vi "Main.vi"() -> ()   [LabVIEW 2013]
doc: "Main code that will run on the robot and contains all the logic and hardware interfaces."
uses:
  Data/TypeDefs/UTM Location.ctl
  Data/TypeDefs/Sail Set Suggestions.ctl
  Data/TypeDefs/Rudder Set Suggestions.ctl
  Data/TypeDefs/OverrideInformation.ctl
  Data/TypeDefs/OverrideMode.ctl
  Logic/Classes/Missions/GenericMission/GenericMission.lvclass
  Logic/Classes/Obstacle/Obstacle.lvclass
  Logic/Classes/Logger/Logger.lvclass
panel:
  out "appended path":path
  out "Missions":refnum<class "GenericMission.lvclass">[](array[class])
  out "Obstacles":refnum<class "Obstacle.lvclass">[](array[class])
  out "Finished Missions":refnum<class "GenericMission.lvclass">[](array[class])
  out "OverrideInformation":T1={"OverrideMode"=enum."Rudder", "SailSetting"={"MainSailSuggestion"=0.0, "JibSailSuggestion"=0.0}, "Rudder Setpoint"=0.0, "Sim_Wind_Speed"=0.0, "Sim_Wind_Heading"=0.0} {"SailSetting"."MainSailSuggestion" min=0.0 max=1.0; "SailSetting"."JibSailSuggestion" min=0.0 max=1.0; "Rudder Setpoint" min=-0.95 max=0.95 scale=1.0..-1.0}
  out "DisplayCounter":i32
  out "AbsWindDirection":dbl
  out "IronsRange":dbl
  out "RudderPosition":T4 min=-0.95 max=0.95 scale=1.0..-1.0
  out "SailPositions":T3 {"MainSailSuggestion" min=0.0 max=1.0; "JibSailSuggestion" min=0.0 max=1.0}
  out "RelWindDirection":dbl
  out "RateOfTurn":dbl
  out "BoatLocation":T5 {"North" format="%#_10f"; "East" format="%#_8f"}
  out "BoatDirection":dbl
  out "WindSpeed":dbl
  out "BoatSpeed":dbl
  in  "XBee Serial Port":refnum<visa-resource-name>="COM8"
  in  "Boat Type":T6(ring)=enum."Simulation"
  in  "stop":bool
  # "ALL THE DEBUG INFO - Eric"
  # "SET THIS BEFORE RUNNING\nOR YOU WILL NEED TO\nRESTART THE CODE!!!"
  # "For Little Boat Initialization"
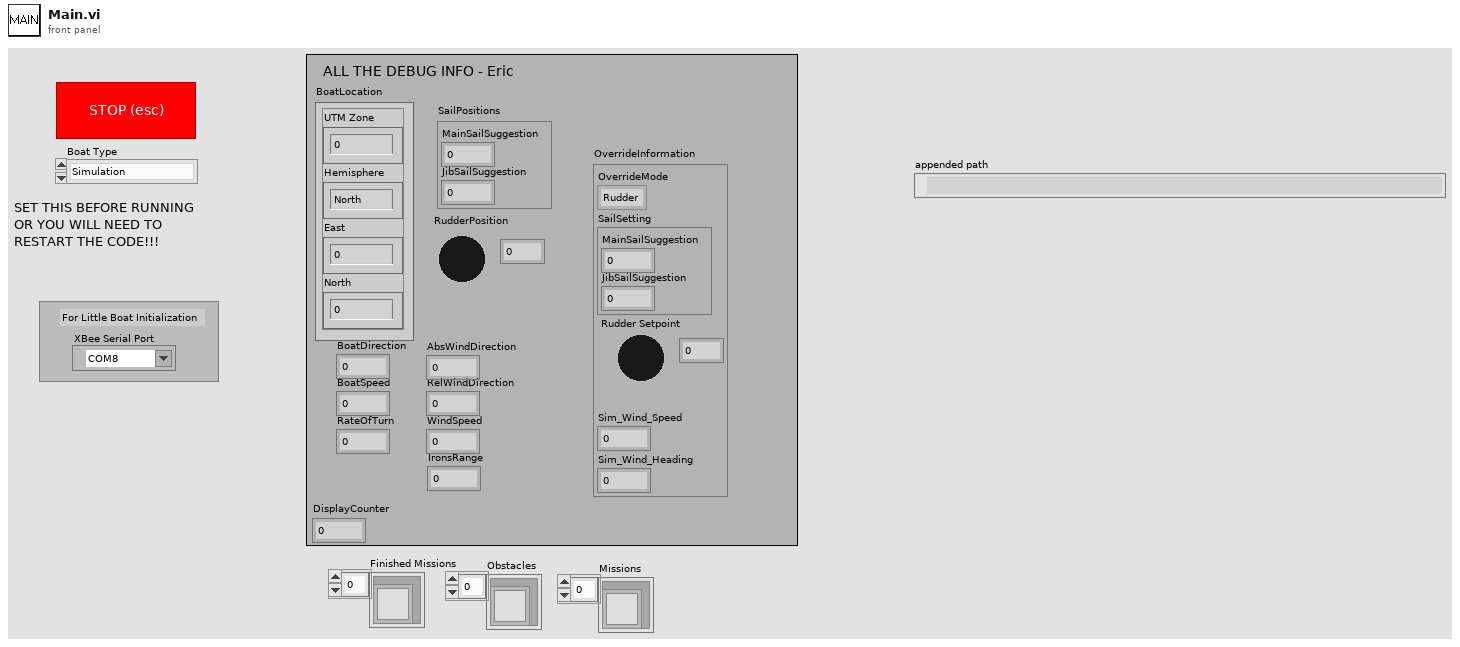
[diagram p1: front panel]
types:
  T1 = typedef "OverrideInformation.ctl" = cluster{"OverrideMode":T2, "SailSetting":T3, "Rudder Setpoint":T4, "Sim_Wind_Speed":dbl, "Sim_Wind_Heading":dbl}
  T2 = typedef "OverrideMode.ctl" = enum16{"None", "Rudder", "Sails", "Both"}
  T3 = typedef "Sail Set Suggestions.ctl" = cluster{"MainSailSuggestion":dbl, "JibSailSuggestion":dbl}
  T4 = typedef "Rudder Set Suggestions.ctl" = dbl
  T5 = typedef "UTM Location.ctl" = cluster{"UTM Zone":dbl, "Hemisphere":enum16{"North", "South"}, "East":dbl, "North":dbl}
  T6 = enum16{"Blackbody Radiation", "Little boats", "Simulation", "Damn Yankee"}
  T7 = typedef "MissionNotifiers.ctl" = cluster{"Missions":refnum<notifier>, "Finished Missions":refnum<notifier>, "Obstacles":refnum<notifier>}
  T8 = typedef "Notifiers.ctl" = cluster{"BoatSpeed":refnum<notifier>, "WindSpeed":refnum<notifier>, "EStop":refnum<notifier>, "BoatDirection":refnum<notifier>, "Luffing":refnum<notifier>, "RudderForce":refnum<notifier>, "BatteryVoltage":refnum<notifier>, "StayForces":refnum<notifier>, "BoatLocation":refnum<notifier>, "Pitch":refnum<notifier>, "Roll":refnum<notifier>, "RateOfTurn":refnum<notifier>, "RelWindDirection":refnum<notifier>, "SailPositions":refnum<notifier>, "RudderPosition":refnum<notifier>, "IronsRange":refnum<notifier>, "AbsWindDirection":refnum<notifier>, "OverrideInformation":refnum<notifier>, "DynamixelTorques":refnum<notifier>, "MotorSetup":refnum<notifier>, "AirmarStatus":refnum<notifier>, "HardwareOnline?":refnum<notifier>, "Sim_ActualSailPositions [0,1]":refnum<notifier>, "DynamixelCycleTracker":refnum<notifier>, "BoatVelocityDirection":refnum<notifier>, "SimWindHeading(rad)":refnum<notifier>, "SimWindSpeed(m/s)":refnum<notifier>, "RCInputValues":refnum<notifier>, "Finished Waypoints":refnum<notifier>, "DesiredHeading":refnum<notifier>, "Latest Mission ID":refnum<notifier>, "Latest Obstacle ID":refnum<notifier>}
  T9 = typedef "Queues.ctl" = cluster{"Waypoints":refnum<queue>}
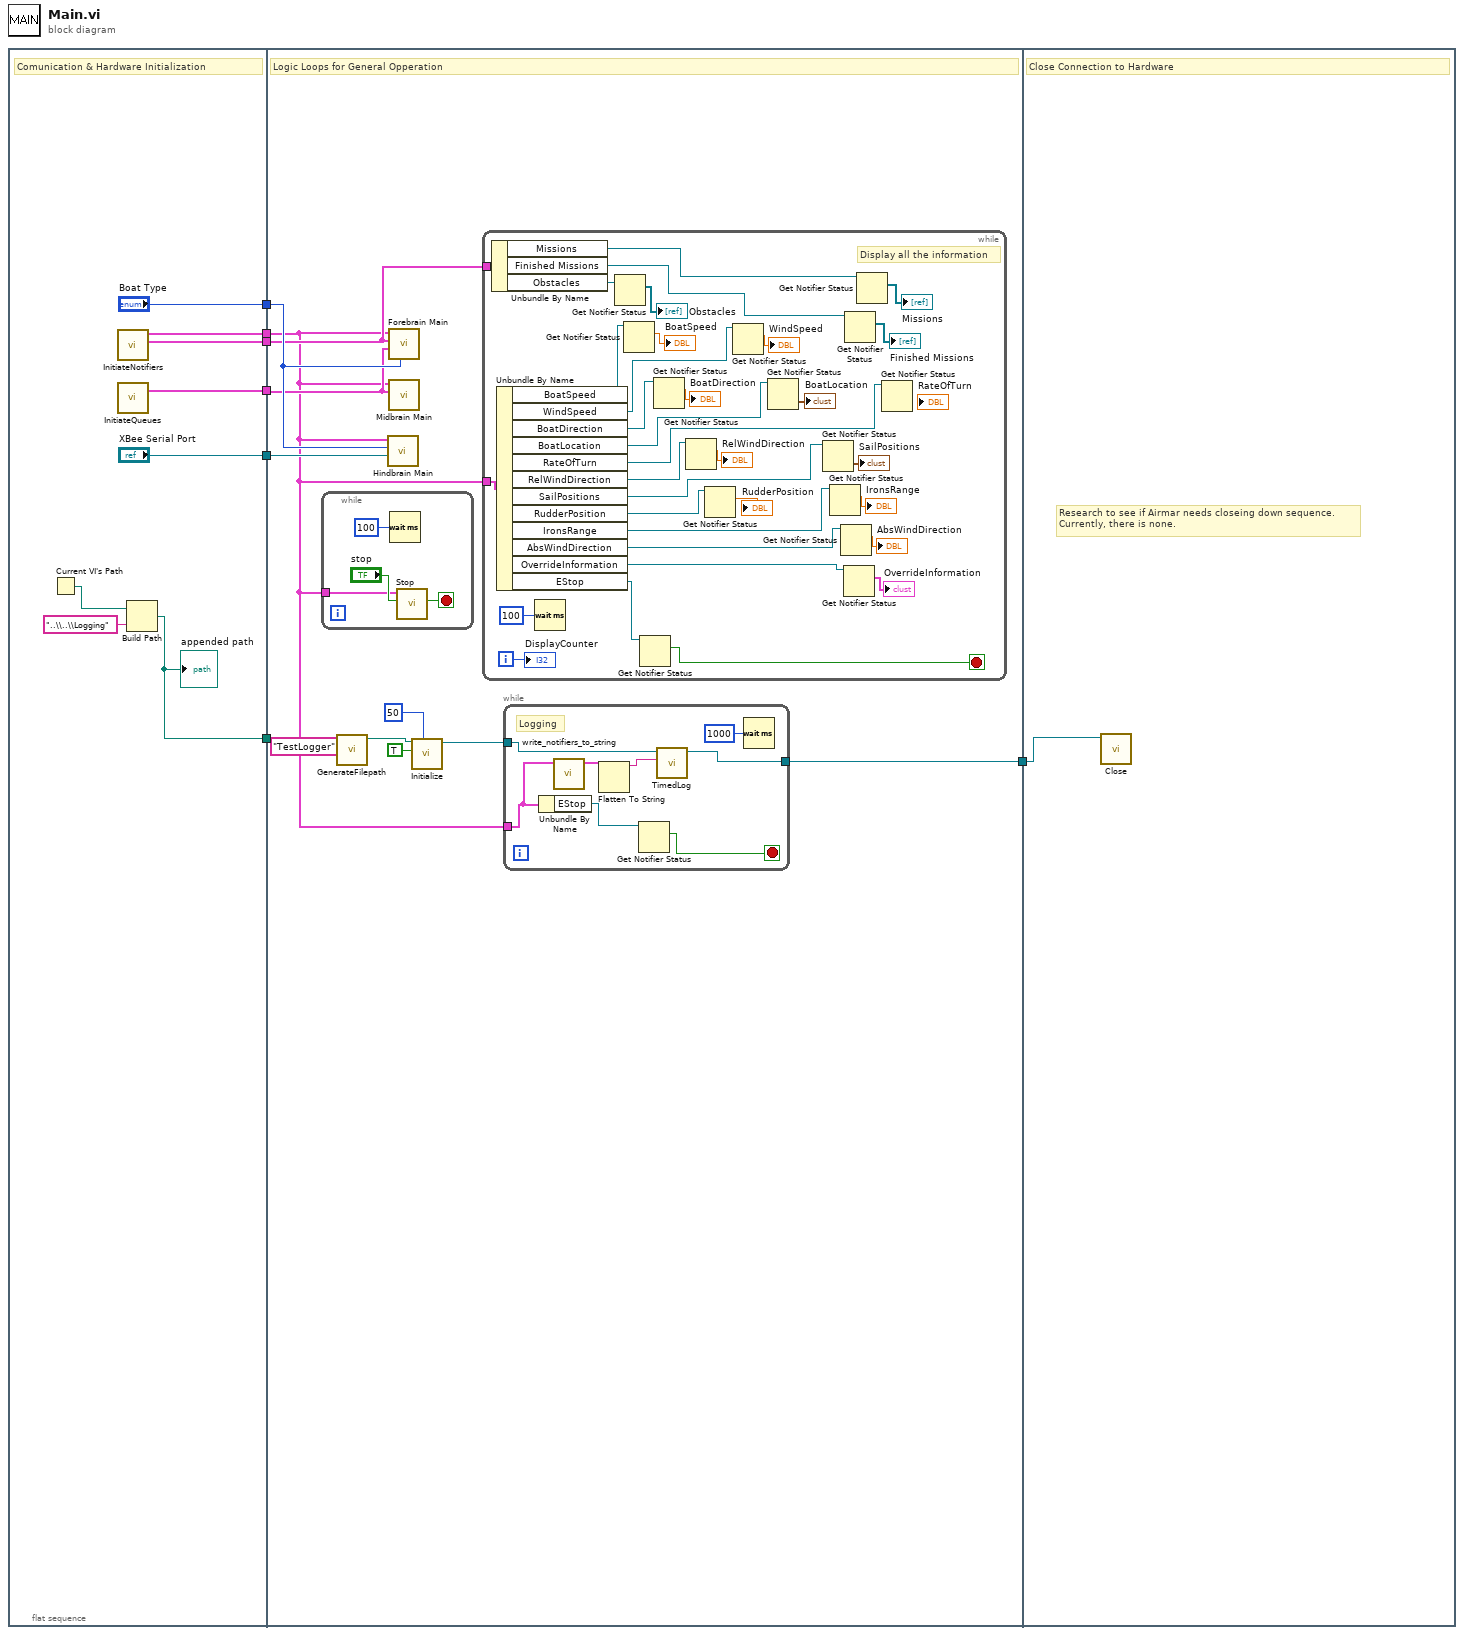
[diagram p0: block diagram]
diagram:
  n1 = flat-sequence {
    tunnel: [w15] -> w7
    tunnel: ["Boat Type"] -> w6
    tunnel: [w13] -> w5
    tunnel: ["XBee Serial Port"] -> w4
    tunnel: [w11] -> w3
    tunnel: [w8] -> w1
    tunnel: w7 -> [w25]
    tunnel: w6 -> [w26]
    tunnel: w5 -> [w23]
    tunnel: w4 -> [w27]
    tunnel: w3 -> [w24]
    tunnel: [w18] -> w2
    tunnel: w1 -> [w16]
    tunnel: w2 -> [w73]
    frame #0 {
      # "Comunication & Hardware Initialization"
      n2 = Current VI's Path() -> (path=w10:path)
      n3 = call "InitiateNotifiers.vi"() -> ("Mission Notifiers"=w11:T7, "NotifierReferences"=w13:T8)  [unwired: 9 in, 1 out]
      n4 = call "InitiateQueues.vi"() -> ("Queue References"=w15:T9)  [unwired: 3 in]
      n5 = Build Path(base path=w10, name or relative path="..\\..\\Logging") -> (appended path=w8:path)
      "appended path" <- w8
    }
    frame #1 {
      # "Logic Loops for General Opperation"
      n6 = while {
        tunnel: w23 -> [w69]
        stop <- w70 stop-if-true
        n7 = Wait (ms)(milliseconds to wait=u32 100) -> ()  [unwired: 1 out]
        n8 = call "Stop.vi"("StopButton"="stop", "NotifierReff"=w69) -> ("StopOut"=w70:bool)  [unwired: 9 in]
      }
      n9 = call "GenerateFilepath.vi"("Identifier"="TestLogger", "Data storage folder"=w16) -> ("File path out"=w19:path)  [unwired: 8 in, 1 out]
      n10 = call "Hindbrain Main.vi"("XBee Serial Port"=w27, "Boat Type"=w26, "NotifierReff"=w23) -> ()  [unwired: 9 in]
      n11 = call "Forebrain Main.vi"("Boat Type"=w26, "QueueRef"=w25, "Mission Notifiers"=w24, "NotifierReff"=w23) -> ()  [unwired: 7 in, 1 out]
      n12 = call "Midbrain Main.vi"("Waypoint Queue Ref"=w25, "Notifier Ref"=w23) -> ()  [unwired: 10 in]
      n13 = call "Initialize.vi"("buffer size"=50, "Enable? (T)"=TRUE, "File path"=w19) -> ("Logger out"=w20:refnum<class "Logger.lvclass">)  [unwired: 7 in, 1 out]
      n14 = while {
        tunnel: w23 -> [w67]
        tunnel: w24 -> [w42]
        i -> [w47]
        stop <- w44 stop-if-true
        # "Display all the information"
        n15 = Unbundle By Name(w42) -> ("Missions"=w37:refnum<notifier>, "Finished Missions"=w39:refnum<notifier>, "Obstacles"=w41:refnum<notifier>)
        n16 = Unbundle By Name(w67) -> ("BoatSpeed"=w66:refnum<notifier>, "WindSpeed"=w64:refnum<notifier>, "BoatDirection"=w61:refnum<notifier>, "BoatLocation"=w60:refnum<notifier>, "RateOfTurn"=w58:refnum<notifier>, "RelWindDirection"=w56:refnum<notifier>, "SailPositions"=w55:refnum<notifier>, "RudderPosition"=w53:refnum<notifier>, "IronsRange"=w50:refnum<notifier>, "AbsWindDirection"=w48:refnum<notifier>, "OverrideInformation"=w46:refnum<notifier>, "EStop"=w43:refnum<notifier>)
        n17 = Wait (ms)(milliseconds to wait=u32 100) -> ()  [unwired: 1 out]
        n18 = Get Notifier Status(notifier=w41) -> (current notification=→"Obstacles":refnum<class "Obstacle.lvclass">[])  [unwired: 1 in, 4 out]
        n19 = Get Notifier Status(notifier=w66) -> (current notification=→"BoatSpeed":dbl)  [unwired: 1 in, 4 out]
        n20 = Get Notifier Status(notifier=w43) -> (current notification=w44:bool)  [unwired: 1 in, 4 out]
        n21 = Get Notifier Status(notifier=w61) -> (current notification=→"BoatDirection":dbl)  [unwired: 1 in, 4 out]
        n22 = Get Notifier Status(notifier=w56) -> (current notification=→"RelWindDirection":dbl)  [unwired: 1 in, 4 out]
        n23 = Get Notifier Status(notifier=w53) -> (current notification=→"RudderPosition":T4)  [unwired: 1 in, 4 out]
        n24 = Get Notifier Status(notifier=w64) -> (current notification=→"WindSpeed":dbl)  [unwired: 1 in, 4 out]
        n25 = Get Notifier Status(notifier=w60) -> (current notification=→"BoatLocation":T5)  [unwired: 1 in, 4 out]
        n26 = Get Notifier Status(notifier=w55) -> (current notification=→"SailPositions":T3)  [unwired: 1 in, 4 out]
        n27 = Get Notifier Status(notifier=w50) -> (current notification=→"IronsRange":dbl)  [unwired: 1 in, 4 out]
        n28 = Get Notifier Status(notifier=w48) -> (current notification=→"AbsWindDirection":dbl)  [unwired: 1 in, 4 out]
        n29 = Get Notifier Status(notifier=w46) -> (current notification=→"OverrideInformation":T1)  [unwired: 1 in, 4 out]
        n30 = Get Notifier Status(notifier=w39) -> (current notification=→"Finished Missions":refnum<class "GenericMission.lvclass">[])  [unwired: 1 in, 4 out]
        n31 = Get Notifier Status(notifier=w37) -> (current notification=→"Missions":refnum<class "GenericMission.lvclass">[])  [unwired: 1 in, 4 out]
        n32 = Get Notifier Status(notifier=w58) -> ()  [unwired: 1 in, 5 out]
        "DisplayCounter" <- w47
      }
      n33 = while {
        tunnel: w23 -> [w30]
        tunnel: w20 -> [w32]
        tunnel: [w31] -> w18
        stop <- w34 stop-if-true
        # "Logging"
        n34 = Unbundle By Name(w30) -> ("EStop"=w35:refnum<notifier>)
        n35 = call "write_notifiers_to_string.vi"("NotifierReff"=w30) -> ("input cluster"=w28:cluster{"names":string, "value":variant})  [unwired: 10 in]
        n36 = Flatten To String(anything=w28) -> (data string=w29:string)  [unwired: 3 in, 2 out]
        n37 = Get Notifier Status(notifier=w35) -> (current notification=w34:bool)  [unwired: 1 in, 4 out]
        n38 = call "TimedLog.vi"("Message"=w29, "Logger in"=w32) -> ("Logger out"=w31:refnum<class "Logger.lvclass">)  [unwired: 7 in, 2 out]
        n39 = Wait (ms)(milliseconds to wait=u32 1000) -> ()  [unwired: 1 out]
      }
    }
    frame #2 {
      # "Research to see if Airmar needs closeing down sequence.\nCurrently, there is none."
      # "Close Connection to Hardware"
      n40 = call "Close.vi"("Logger in"=w73) -> ()  [unwired: 10 in, 1 out]
    }
  }
